vi "Iterate.vi"(10 "Iterate":i32, 11 "Hello World Event in":refnum<class "Hello World Event.lvclass">) -> (3 "Hello World Event out":refnum<class "Hello World Event.lvclass">)   [LabVIEW 2021, in "Hello World Event.lvlib" / "Hello World Event.lvclass"]
uses:
  Hello World Event.lvclass
  Hello World Event.lvclass/Hello World Event.ctl
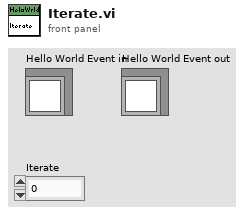
[diagram p1: front panel]
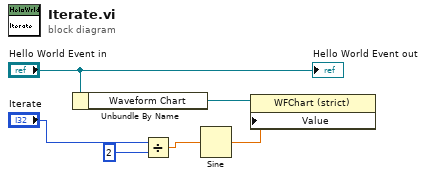
[diagram p0: block diagram]
diagram:
  n1 = Unbundle By Name("Hello World Event in") -> ("Waveform Chart"=w5:refnum<vi>)
  n2 = Divide(x="Iterate", y=2) -> (x/y=w2:dbl)
  n3 = Sine(x=w2) -> (sin(x)=w3:dbl)
  n4 = property class="WFChart (strict)"(reference=w5, "Value"=w3) -> ()  [unwired: 1 in, 2 out]
  "Hello World Event out" <- "Hello World Event in"
